vi "PPMS Global.vi"() -> ()   [LabVIEW 2016, in "instrument.PPMS2.lvclass"]
uses:
  instrument.PPMS2.lvclass
panel:
  out "Field Status":i32(ring)=1 items=["MagnetUnknown"=0, "StablePersistent"=1, "WarmingSwitch"=2, "CoolingSwitch"=3, "StableDriven"=4, "Iterating"=5, "Charging"=6, "Discharging"=7, "CurrentError"=8, "MagnetFailure"=15]
  out "Temperature Status":T1(ring)=enum."Stable"
  out "Helium Level String":string
  out "Helium Level":dbl=100.0
  out "Rate (K/min)":dbl=5.0
  out "Rate (Oe/s)":dbl=10.0
  out "Target Position":dbl
  out "Target Temp":dbl
  out "Target Field":dbl
  out "Set Position?":bool
  out "Set Temp?":bool
  out "Set Field?":bool
  out "Position (Degree)":dbl=-0.001072365790605545 format="%#.3g"
  out "PPMS IP Address":string="130.49.180.87"
  out "Field (Oe)":dbl=-0.001072365790605545 format="%#.3g"
  out "Temperature (K)":dbl=309.9967
  # "PPMS2 Global Variables"
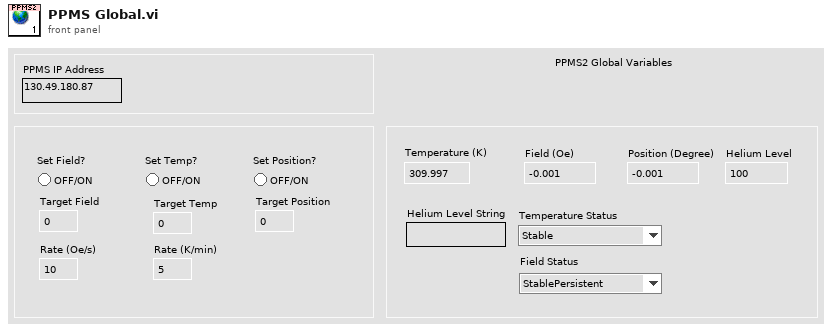
[diagram p1: front panel]
types:
  T1 = enum16{"TemperatureUnknown", "Stable", "Tracking", "Near", "Chasing", "Filling", "Standby", "Disabled", "ImpedanceNotFunction", "TempFailure"}
diagram:
